vi "servo smooth.vi"(7 "Servo Number":u8, 8 "等待时间（毫秒）":u32=30, 9 "手臂当前值输入":u8, 10 "servo In":u8, 11 "Arduino Resource":T1) -> (1 "手臂当前值输出":u8, 3 "Arduino Resource out":T1={"VISA resource"="", "Board Type"=enum."Uno", "Connection Type"=enum."USB / Serial", "Bytes Per Packet (15)"=15})   [LabVIEW 2016]
uses:
  <vilib>/LabVIEW Interface for Arduino/Type Defs/Arduino Resource.ctl
  <vilib>/LabVIEW Interface for Arduino/Type Defs/Board Type.ctl
  <vilib>/LabVIEW Interface for Arduino/LabVIEW Interface for Arduino.lvlib
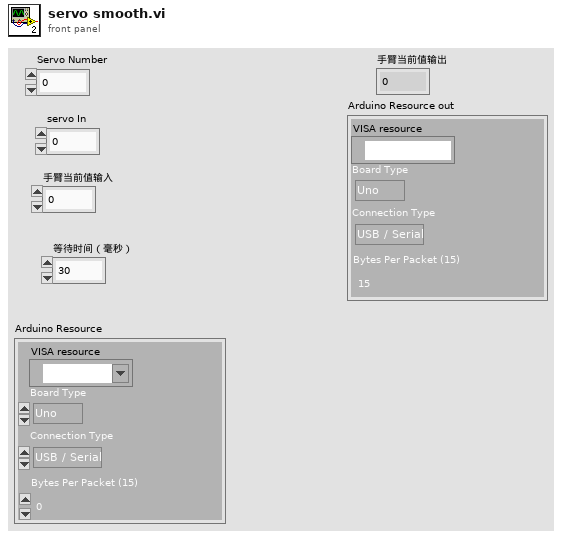
[diagram p1: front panel]
types:
  T1 = typedef "LabVIEW Interface for Arduino.lvlib/Arduino Resource.ctl" = cluster{"VISA resource":refnum<visa-resource-name>, "Board Type":T2, "Connection Type":enum8{"USB / Serial"}, "Bytes Per Packet (15)":u8}
  T2 = typedef "LabVIEW Interface for Arduino.lvlib/Board Type.ctl" = enum16{"Uno", "Dimuelanove w/Atmega 328", "Mega 2560"}
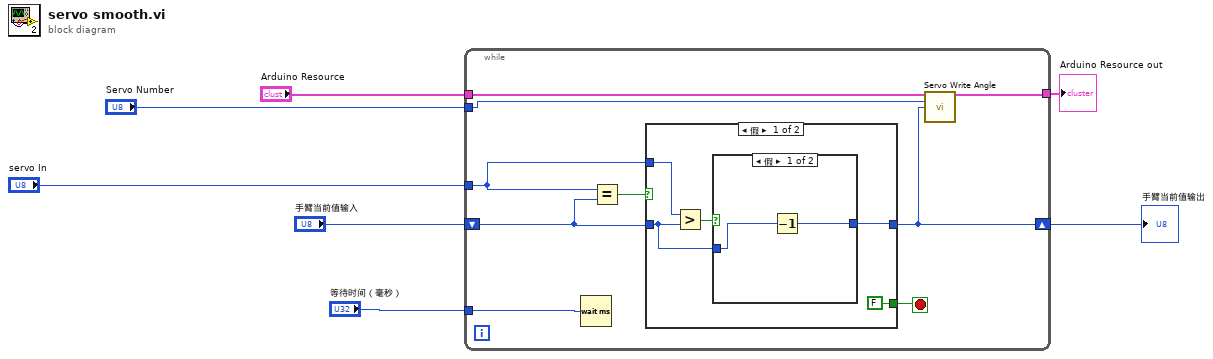
[diagram p0: block diagram]
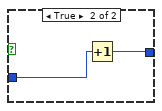
[diagram p2: hidden frame]
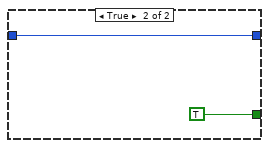
[diagram p3: hidden frame]
diagram:
  n1 = while {
    tunnel: "Arduino Resource" -> [w16]
    shift-right: [w11] -> w6
    shift-left: "手臂当前值输入" -> [w13]
    tunnel: "servo In" -> [w12]
    tunnel: "Servo Number" -> [w10]
    tunnel: "等待时间（毫秒）" -> [w9]
    tunnel: [w8] -> w1
    stop <- w15 stop-if-true
    n2 = Wait (ms)(milliseconds to wait=w9) -> ()  [unwired: 1 out]
    n3 = Equal?(x=w12, y=w13) -> (x = y?=w14:bool)
    n4 = case shown="假" w14 {
      tunnel: [w20 w26] -> w11
      tunnel: [FALSE TRUE] -> w15
      tunnel: w13 -> [w17 w26]
      tunnel: w12 -> [w18 _]
      frame False {
        n5 = Greater?(x=w18, y=w17) -> (0:w21:bool)
        n6 = case shown="假" w21 {
          tunnel: [w23 w25] -> w20
          tunnel: w17 -> [w22 w24]
          frame False {
            n7 = Decrement(x=w22) -> (x-1=w23:u8)
          }
          frame True {
            n8 = Increment(x=w24) -> (x+1=w25:u8)
          }
        }
      }
      frame True {
      }
    }
    n9 = call <vilib>:"Servo Write Angle.vi"("Arduino Resource"=w16, "Servo Number"=w10, "Angle (Degrees)"=w11) -> ("Arduino Resource"=w8:T1)  [unwired: 11 in, 1 out]
  }
  "手臂当前值输出" <- w6
  "Arduino Resource out" <- w1
